vi "RequestInsertSignals_dir.vi"(5 "Signals":T1[](array[typedef]), 11 "error in (no error)":errorcluster) -> (6 "request":string, 15 "error out":errorcluster)   [LabVIEW 2019, in "Logger.lvclass"]
uses:
  Logger.lvclass
  SignalData.ctl
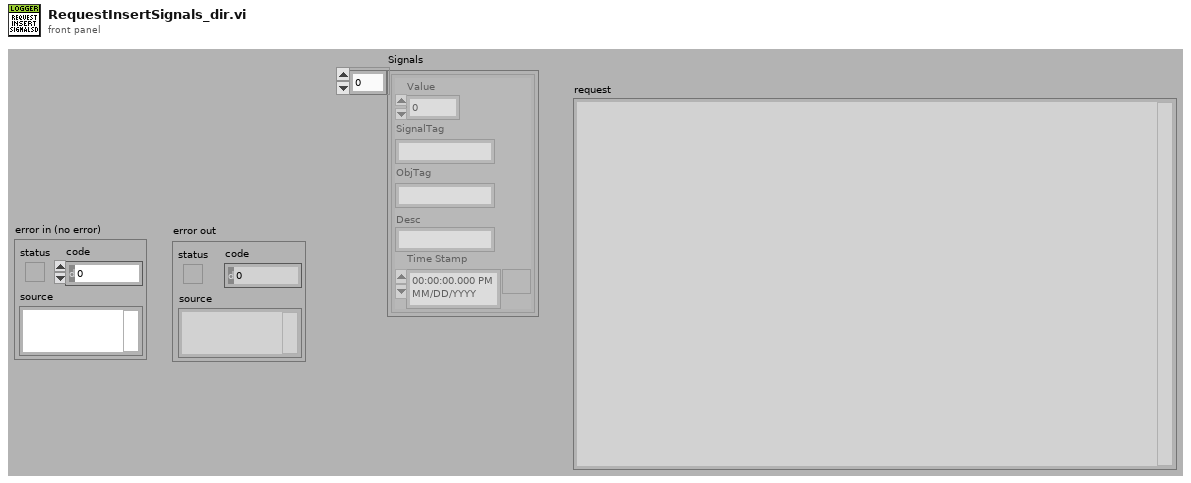
[diagram p1: front panel]
types:
  T1 = typedef "Logger.lvclass/SignalData.ctl" = cluster{"Value":dbl, "SignalTag":string, "ObjTag":string, "Desc":string, "Time Stamp":timestamp}
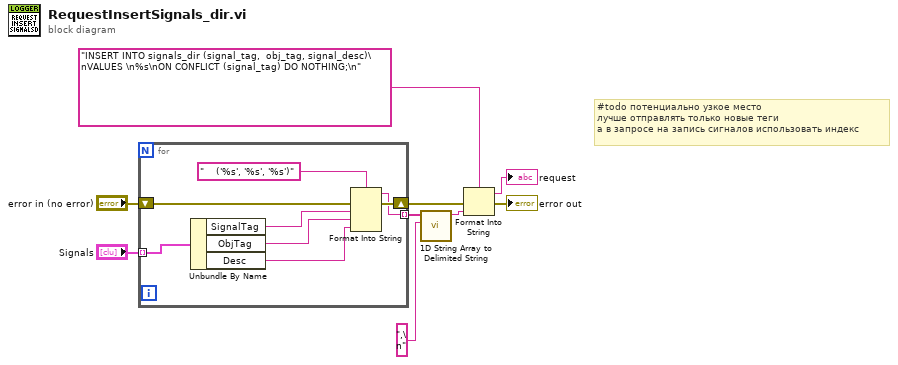
[diagram p0: block diagram]
diagram:
  # "#todo потенциально узкое место\nлучше отправлять только новые теги\nа в запросе на запись сигналов использовать индекс"
  n1 = for {
    tunnel: [w16] -> w8 mode=indexing
    tunnel: "Signals" -> [w13] mode=indexing
    shift-right: [w17] -> w3
    shift-left: "error in (no error)" -> [w15]
    n2 = Unbundle By Name(w13) -> ("SignalTag"=w12:string, "ObjTag"=w11:string, "Desc"=w10:string)
    n3 = Format Into String(format string="    ('%s', '%s', '%s')", error in=w15, w12, w11, w10) -> (resulting string=w16:string, error out=w17:errorcluster)  [unwired: 1 in]
  }
  n4 = call <vilib>:"1D String Array to Delimited String.vi"("delimiter"=",\n", "string array"=w8) -> ("delimited string"=w4:string)  [unwired: 9 in]
  n5 = Format Into String(format string="INSERT INTO signals_dir (signal_tag,  obj_tag, signal_desc)\nVALUES \n%s\nON CONFLICT (signal_tag) DO NOTHING;\n", error in=w3, w4) -> (resulting string=→"request":string, error out=→"error out":errorcluster)  [unwired: 1 in]
